vi "Questionable Temperature Status Query.vi"(0 "VISA resource name":refnum<visa-resource-name>, 11 "error in (no error)":errorcluster) -> (4 "VISA resource name out":refnum<visa-resource-name>, 6 "Questionable Temperature Status":T1, 15 "error out":errorcluster)   [LabVIEW 2018, in "XP Power PLS600.lvlib"]
doc: "Returns the integer data explaining the questionable status monitored in the instrument.\n\nThe Questionable Temperature Status register consists of the following 2 bits:\n\nBit 0: Output Board Over-Temp\nBit 1: Primary Board Over-Temp"
uses:
  XP Power PLS600.lvlib
panel:
  # "Bit 0:  Output Board Over-Temp\nBit 1:  Primary Board Over-Temp"
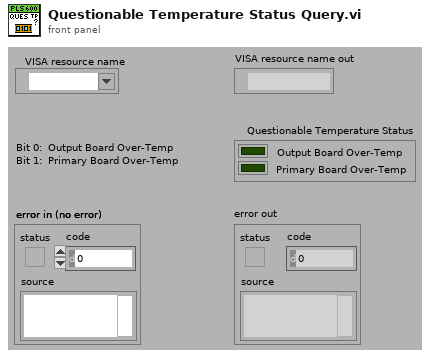
[diagram p1: front panel]
types:
  T1 = cluster{"Output Board Over-Temp":bool, "Primary Board Over-Temp":bool}
  T2 = cluster{"Operation Complete":bool, "Not Used":bool}
  T3 = cluster{"Boolean array[0]":bool, "Boolean array[1]":bool}
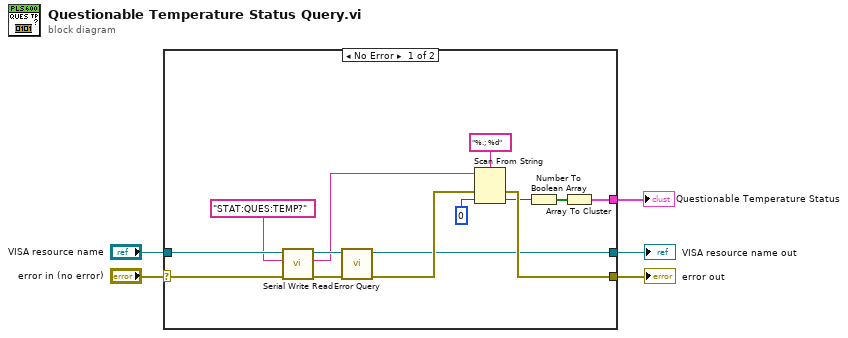
[diagram p0: block diagram]
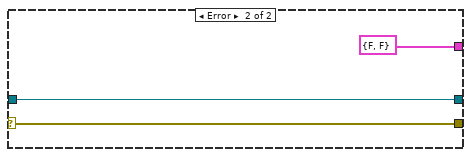
[diagram p2: hidden frame]
diagram:
  n1 = case shown="No Error" "error in (no error)" {
    selector: "error in (no error)" -> [w11 w22]
    tunnel: [w18 w22] -> w5
    tunnel: [w6 w21] -> w4
    tunnel: "VISA resource name" -> [w12 w21]
    tunnel: [w15 T2 {"Operation Complete"=FALSE, "Not Used"=FALSE} ("Operation Status")] -> w1
    frame No Error {
      n2 = call "Serial Write Read.vi"("error in (no error)"=w11, "Write Buffer"="STAT:QUES:TEMP?" ("Command to Send (empty)"), "VISA resource name"=w12) -> ("error out"=w9:errorcluster, "Read Buffer"=w8:string, "VISA resource name out"=w13:refnum<visa-resource-name>)  [unwired: 6 in]
      n3 = call "Error Query.vi"("error in (no error)"=w9, "VISA resource name"=w13) -> ("error out"=w7:errorcluster, "VISA resource name out"=w6:refnum<visa-resource-name>)  [unwired: 6 in, 2 out]
      n4 = Scan From String(format string="%.; %d" ("Format String"), input string=w8, error in=w7, default 1=u16 0 ("default value 1")) -> (error out=w18:errorcluster, output 1=w14:u16)  [unwired: 1 in, 2 out]
      n5 = Number To Boolean Array(number=w14) -> (Boolean array=w17:bool[])
      n6 = Array To Cluster(array=w17) -> (cluster=w15:T3)
    }
    frame Error {
    }
  }
  "error out" <- w5
  "VISA resource name out" <- w4
  "Questionable Temperature Status" <- w1
